vi "final16_with_sequence.vi"() -> ()   [LabVIEW 2019]
uses:
  <vilib>/Instr/_visa.llb/VISA Configure Serial Port (Instr).vi
  <vilib>/Utility/file.llb/Write Delimited Spreadsheet (DBL).vi
  <vilib>/Analysis/NI_AALPro.lvlib
  <vilib>/Analysis/NI_AALBase.lvlib
panel:
  out "initialized array":dbl[](array[numeric])
  out "standard deviation":dbl format="%0.2f"
  out "variance":dbl format="%0.2f"
  out "mean":dbl format="%0.2f"
  out "Conversion [g]":dbl
  out "slope_gain0":dbl
  out "intercept_gain0":dbl
  out "slope_gain2":dbl
  out "intercept_gain2":dbl
  out "slope_gain1":dbl
  out "intercept_gain1":dbl
  out "Debug array":string[](array[string])
  in  "Stop":bool
  in  "Cycles":dbl min=1.0 step=1.0
  in  "Start operation":bool
  out "String passed to Arduino":string
  in  "Function":u16(ring) items=["Read data ", "Compare different gains", "Execute calibration"]
  out "Received data":string
  in  "Gain":u16(ring) items=["32", "64", "128"]
  in  "Save data path":path
  in  "Arduino COM port":refnum<visa-resource-name>="COM6"
  # "Select all options, then press \"Start operation\" button"
  # "Nerd zone"
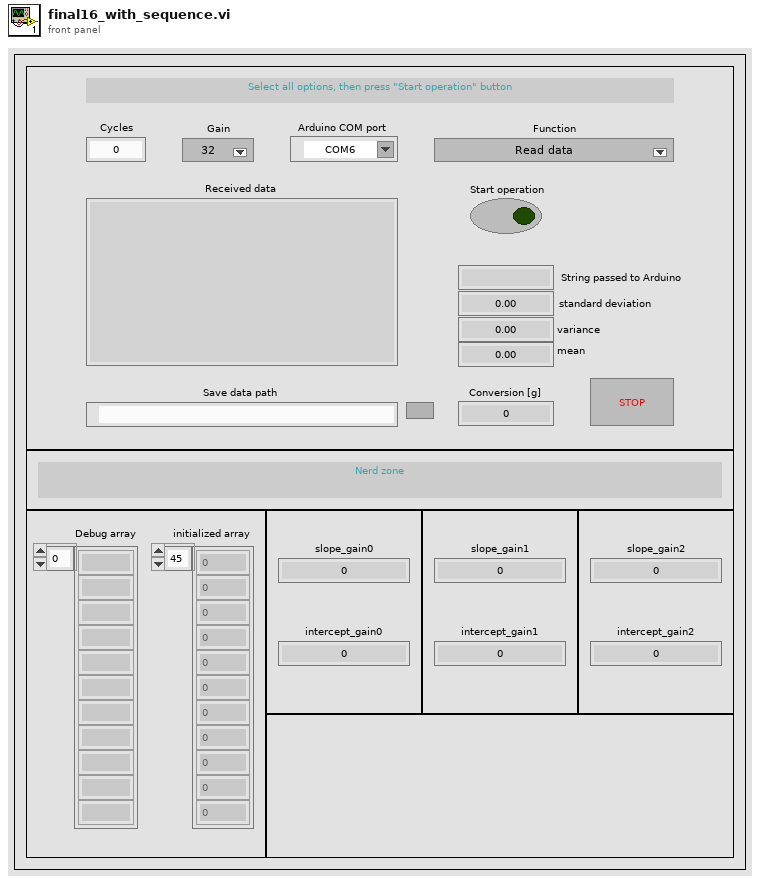
[diagram p1: front panel]
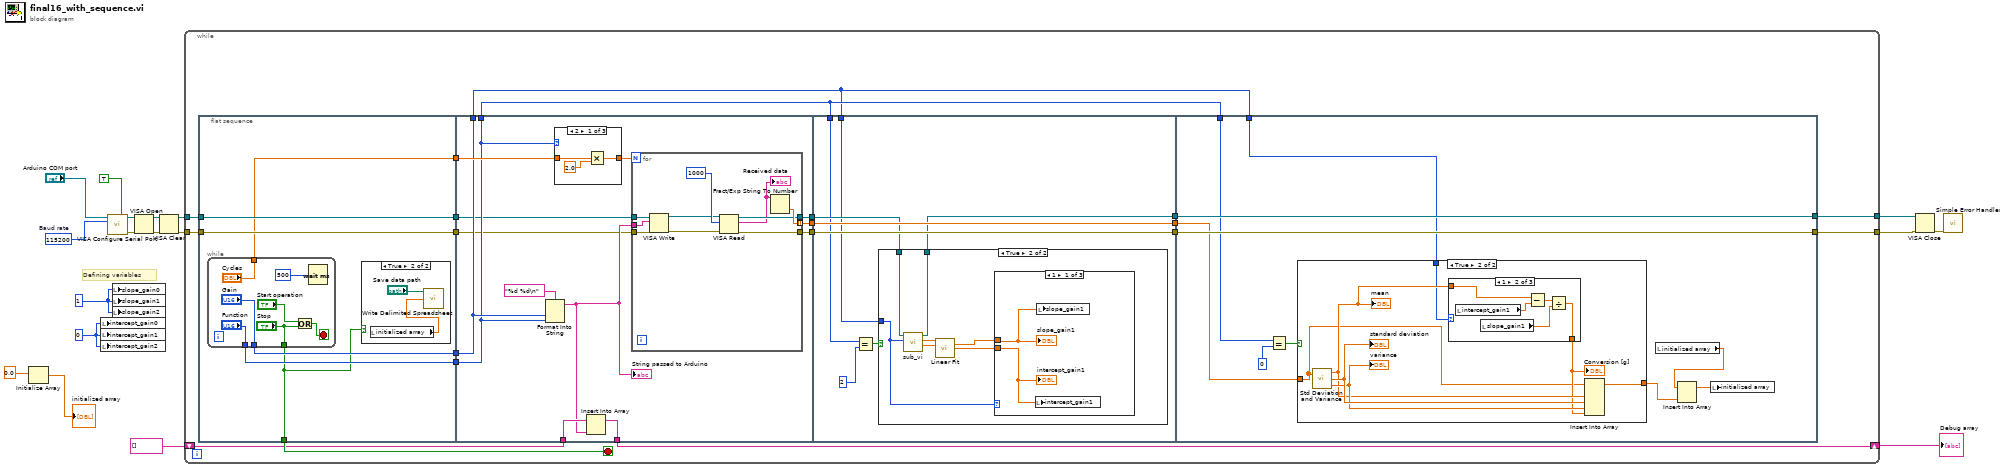
[diagram p0: block diagram]
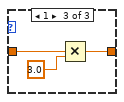
[diagram p4: hidden frame]
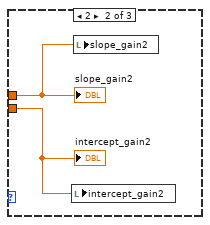
[diagram p6: hidden frame]
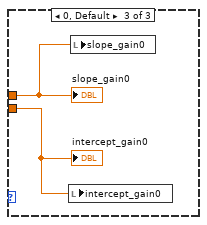
[diagram p7: hidden frame]
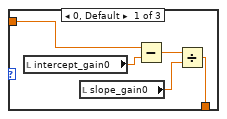
[diagram p9: hidden frame]
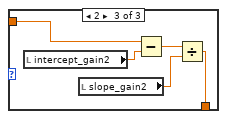
[diagram p10: hidden frame]
diagram:
  w5 = 0
  w4 = 1
  w17 = u32 115200  # Baud rate
  # "Defining variables"
  n1 = Initialize Array(0.0) -> (→"initialized array":dbl[])  [unwired: 1 in]
  n2 = local write "intercept_gain0"(w5) -> ()
  n3 = local write "intercept_gain1"(w5) -> ()
  n4 = local write "intercept_gain2"(w5) -> ()
  n5 = call-poly "VISA Configure Serial Port"("VISA resource name"="Arduino COM port", "Enable Termination\nChar (T)"=TRUE ("Enable Termination\nChar (T)"), "baud rate (9600)"=w17) -> ("VISA resource name out"=w15:refnum<visa-resource-name>, "error out"=w16:errorcluster)  [unwired: 11 in]
  n6 = local write "slope_gain0"(w4) -> ()
  n7 = local write "slope_gain1"(w4) -> ()
  n8 = local write "slope_gain2"(w4) -> ()
  n9 = VISA Open(error in (no error)=w16, VISA resource name=w15) -> (VISA resource name=w12:refnum<visa-resource-name>, error out=w13:errorcluster)  [unwired: 3 in]
  n10 = VISA Clear(VISA resource name=w12, error in (no error)=w13) -> (VISA resource name out=w10:refnum<visa-resource-name>, error out=w11:errorcluster)
  n11 = while {
    tunnel: w11 -> [w38]
    tunnel: w10 -> [w37]
    shift-right: [w36] -> w8
    shift-left: string[] [] -> [w34]
    tunnel: [w20] -> w6
    tunnel: [w19] -> w1
    stop <- w35 stop-if-true
    n12 = flat-sequence {
      tunnel: [w44] -> w33
      tunnel: [w43] -> w32
      tunnel: [w42] -> w31
      tunnel: [w41] -> w30
      tunnel: [w40] -> w29
      tunnel: [w39] -> w35
      tunnel: w37 -> [w43]
      tunnel: w38 -> [w44]
      tunnel: w33 -> [w54]
      tunnel: w32 -> [w55]
      tunnel: w31 -> [w57]
      tunnel: w30 -> [w58]
      tunnel: w29 -> [w61]
      tunnel: [w59] -> w36
      tunnel: w34 -> [w60]
      tunnel: [w66] -> w28
      tunnel: [w65] -> w27
      tunnel: [w64] -> w26
      tunnel: [w58] -> w21
      tunnel: [w57] -> w22
      tunnel: w28 -> [w87]
      tunnel: w27 -> [w91]
      tunnel: w26 -> [w90]
      tunnel: [w91] -> w25
      tunnel: [w90] -> w24
      tunnel: [w86] -> w23
      tunnel: w21 -> [w85]
      tunnel: w22 -> [w84]
      tunnel: [w114] -> w20
      tunnel: [w115] -> w19
      tunnel: w25 -> [w115]
      tunnel: w24 -> [w106]
      tunnel: w23 -> [w114]
      tunnel: w22 -> [w111]
      tunnel: w21 -> [w110]
      frame #0 {
        n13 = while {
          tunnel: ["Function"] -> w42
          tunnel: ["Gain"] -> w41
          tunnel: ["Cycles"] -> w40
          tunnel: ["Stop"] -> w39
          stop <- w48 stop-if-true
          n14 = Or(x="Start operation", y="Stop") -> (x .or. y?=w48:bool)
          n15 = Wait (ms)(milliseconds to wait=u32 500) -> ()  [unwired: 1 out]
        }
        n16 = case shown="True" w39 {
          frame False {
          }
          frame True {
            n17 = local read "initialized array"() -> (w45:dbl[])
            n18 = call-poly <vilib>:"Write Delimited Spreadsheet.vi"("file path (dialog if empty)"="Save data path", "1D data"=w45) -> ()  [unwired: 12 in, 2 out]
          }
        }
      }
      frame #1 {
        n19 = Format Into String(format string="%d %d\n", w58, w57) -> (resulting string=w56:string)  [unwired: 2 in, 1 out]
        "String passed to Arduino" <- w56
        n20 = case shown="2" w57 {
          tunnel: w61 -> [w69 w70 w71]
          tunnel: [w67 w70 w72] -> w62
          frame 2 {
            n21 = Multiply(x=w69, y=2.0) -> (x*y=w67:dbl)
          }
          frame 0, Default {
          }
          frame 1 {
            n22 = Multiply(x=w71, y=3.0) -> (x*y=w72:dbl)
          }
        }
        n23 = Insert Into Array(array=w60, new element=w56) -> (w59:string[])  [unwired: 1 in]
        n24 = for {
          N: w62 -> [_]
          tunnel: [w82] -> w64 mode=indexing
          tunnel: [w81] -> w66
          tunnel: [w83] -> w65
          tunnel: w56 -> [w78]
          tunnel: w55 -> [w75]
          tunnel: w54 -> [w74]
          n25 = VISA Write(VISA resource name=w75, write buffer=w78, error in (no error)=w74) -> (VISA resource name out=w76:refnum<visa-resource-name>, error out=w77:errorcluster)  [unwired: 1 out]
          n26 = VISA Read(VISA resource name=w76, byte count=u32 1000, error in (no error)=w77) -> (VISA resource name out=w81:refnum<visa-resource-name>, read buffer=w80:string, error out=w83:errorcluster)  [unwired: 1 out]
          "Received data" <- w80
          n27 = Fract/Exp String To Number(string=w80) -> (number=w82:dbl)  [unwired: 3 in, 1 out]
        }
      }
      frame #2 {
        n28 = Equal?(x=w84, y=u16 2) -> (x = y?=w88:bool)
        n29 = case shown="True" w88 {
          tunnel: [w92 w98] -> w86
          tunnel: w87 -> [w92 w95]
          tunnel: w85 -> [_ w94]
          frame False {
          }
          frame True {
            n30 = call "sub_vi.vi"("Gain"=w94, "VISA resource name"=w95) -> ("Weights"=w99:dbl[], "Measures"=w93:dbl[], "VISA resource name out"=w98:refnum<visa-resource-name>)  [unwired: 6 in, 1 out]
            n31 = call <vilib>:"Linear Fit.vi"("Y"=w93, "X"=w99) -> ("slope"=w97:dbl, "intercept"=w96:dbl)  [unwired: 9 in, 3 out]
            n32 = case shown="1" w94 {
              tunnel: w97 -> [w101 w103 w105]
              tunnel: w96 -> [w100 w102 w104]
              frame 1 {
                n33 = local write "intercept_gain1"(w100) -> ()
                n34 = local write "slope_gain1"(w101) -> ()
                "slope_gain1" <- w101
                "intercept_gain1" <- w100
              }
              frame 2 {
                n35 = local write "intercept_gain2"(w102) -> ()
                n36 = local write "slope_gain2"(w103) -> ()
                "slope_gain2" <- w103
                "intercept_gain2" <- w102
              }
              frame 0, Default {
                n37 = local write "intercept_gain0"(w104) -> ()
                n38 = local write "slope_gain0"(w105) -> ()
                "slope_gain0" <- w105
                "intercept_gain0" <- w104
              }
            }
          }
        }
      }
      frame #3 {
        n39 = Equal?(x=w111, y=u16 0) -> (x = y?=w112:bool)
        n40 = case shown="True" w112 {
          tunnel: w110 -> [_ w119]
          tunnel: w106 -> [w116 w118]
          tunnel: [w116 w117] -> w109
          frame False {
          }
          frame True {
            n41 = call <vilib>:"Std Deviation and Variance.vi"("X"=w118) -> ("mean"=w121:dbl, "standard deviation"=w123:dbl, "variance"=w122:dbl)  [unwired: 1 in]
            "standard deviation" <- w123
            "variance" <- w122
            "mean" <- w121
            n42 = case shown="1" w119 {
              tunnel: w121 -> [w128 w131 w136]
              tunnel: [w126 w132 w137] -> w120
              frame 0, Default {
                n43 = local read "intercept_gain0"() -> (w125:dbl)
                n44 = local read "slope_gain0"() -> (w124:dbl)
                n45 = Subtract(x=w128, y=w125) -> (x-y=w127:dbl)
                n46 = Divide(x=w127, y=w124) -> (x/y=w126:dbl)
              }
              frame 1 {
                n47 = local read "intercept_gain1"() -> (w130:dbl)
                n48 = local read "slope_gain1"() -> (w129:dbl)
                n49 = Subtract(x=w131, y=w130) -> (x-y=w133:dbl)
                n50 = Divide(x=w133, y=w129) -> (x/y=w132:dbl)
              }
              frame 2 {
                n51 = local read "intercept_gain2"() -> (w135:dbl)
                n52 = local read "slope_gain2"() -> (w134:dbl)
                n53 = Subtract(x=w136, y=w135) -> (x-y=w138:dbl)
                n54 = Divide(x=w138, y=w134) -> (x/y=w137:dbl)
              }
            }
            "Conversion [g]" <- w120
            n55 = Insert Into Array(array=w118, new element #1=w121, new element #2=w123, new element #3=w122, new element #4=w120) -> (w117:dbl[])  [unwired: 1 in]
          }
        }
        n56 = local read "initialized array"() -> (w108:dbl[])
        n57 = Insert Into Array(array=w108, new element=w109) -> (w107:dbl[])  [unwired: 1 in]
        n58 = local write "initialized array"(w107) -> ()
      }
    }
  }
  "Debug array" <- w8
  n59 = VISA Close(VISA resource name=w6, error in (no error)=w1) -> (error out=w7:errorcluster)
  n60 = call <vilib>:"Simple Error Handler.vi"("error in (no error)"=w7) -> ()  [unwired: 4 in, 5 out]
